vi "libssh2_agent_disconnect - invalid agent - no error 1097.vi"() -> ()   [LabVIEW 2013, in "libssh2_tests.lvlib"]
uses:
  libssh2_tests.lvlib
  libssh2/Agent Refnum.ctl
  libssh2/libssh2_init_default.vi
  <vilib>/Utility/error.llb/General Error Handler.vi
  <vilib>/addons/_JKI Toolkits/Caraya/classes/Assert/Assert.vi
  <vilib>/addons/_JKI Toolkits/Caraya/classes/Assert/Assert Not Error.vi
  libssh2/libssh2.lvlib
  <vilib>/addons/_JKI Toolkits/Caraya/classes/Test/Test.lvclass
panel:
  out "error out":errorcluster
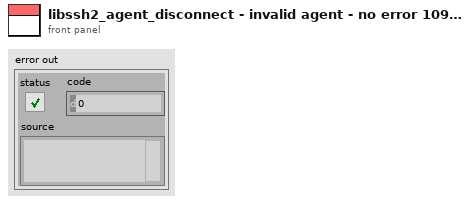
[diagram p1: front panel]
types:
  T1 = typedef "libssh2.lvlib/Agent Refnum.ctl" = refnum<k1>
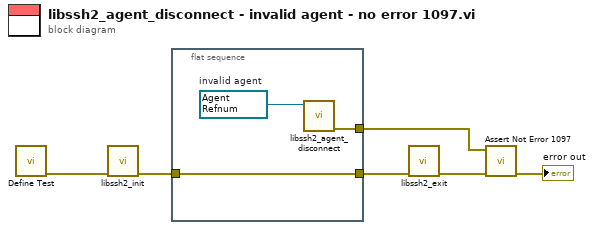
[diagram p0: block diagram]
diagram:
  n1 = call <vilib>:"Define Test.vi"() -> ("error out"=w6:errorcluster)  [unwired: 10 in, 1 out]
  n2 = call-poly "libssh2_init.vi"("error in (no error)"=w6) -> ("error out"=w4:errorcluster)  [unwired: 10 in]
  n3 = flat-sequence {
    tunnel: [w9] -> w3
    tunnel: w4 -> [w9]
    tunnel: [w8] -> w2
    frame #0 {
      w7 = T1 refnum items=["Agent"]  # invalid agent
      n4 = call "libssh2_agent_disconnect.vi"("agent"=w7) -> ("error out"=w8:errorcluster)  [unwired: 10 in]
    }
  }
  n5 = call "libssh2_exit.vi"("error in (no error)"=w3) -> ("error out"=w5:errorcluster)  [unwired: 10 in]
  n6 = call "Assert Not Error 1097.vi"("error in (no error)"=w5, "actual value"=w2) -> ("error out"=→"error out":errorcluster)  [unwired: 9 in]
